vi "Finish.vi"   [LabVIEW 2012]
doc: "This VI is called just before exiting. It is expected to close I/O refnum, save collected data, etc."
uses:
  <vilib>/Rock Robotics/WPI/Joystick/WPI_JoystickGetSetRefNum.vi
  <vilib>/Rock Robotics/WPI/RobotDrive/WPI_RobotDriveGetSetRefNum.vi
types:
  T1 = typedef "WPI_DigitalInputDevRef.ctl" = cluster{"DevStatus":errorcluster, "DIO Channel":T2, "Digital Module":T3}
  T2 = typedef "FPGA_DIOChannel.ctl" = enum8{"DIO 1", "DIO 2", "DIO 3", "DIO 4", "DIO 5", "DIO 6", "DIO 7", "DIO 8", "DIO 9", "DIO 10", "DIO 11", "DIO 12", "DIO 13", "DIO 14", "Invalid"}
  T3 = typedef "FPGA_TypedefDigitalModule.ctl" = enum16{"Digital Module 1", "Digital Module 2"}
  T4 = typedef "WPI_EncoderDevRef.ctl" = cluster{"DevStatus":errorcluster, "EncoderIndex":T5, "CounterIndex":T6, "DistancePerCount":dbl, "Decoding Type":T7}
  T5 = typedef "FPGA_EncoderIdx.ctl" = enum8{"Enc 0", "Enc 1", "Enc 2", "Enc 3", "Invalid"}
  T6 = typedef "FPGA_CounterCtrSystemIndex.ctl" = enum8{"Ctr 0", "Ctr 1", "Ctr 2", "Ctr 3", "Ctr 4", "Ctr 5", "Ctr 6", "Ctr 7", "Invalid"}
  T7 = typedef "WPI_EncoderType.ctl" = enum16{"1x", "2x", "4x"}
  T8 = typedef "WPI_MotorControlDeviceRef.ctl" = cluster{"DeviceStatus":errorcluster, "Type":enum16{"PWM", "CAN"}, "PWM":cluster{"Digital Module":T3, "PWM Channel":T9, "DeadBand":T10}, "CAN":cluster{"Device Number":u8, "Control Mode":T11, "Semaphore":T12, "Max Vout":dbl}, "Invert":bool, "TransformRef":T13, "InvTransformRef":T13}
  T9 = typedef "FPGA_DIOPWMChannel.ctl" = enum8{"PWM 1", "PWM 2", "PWM 3", "PWM 4", "PWM 5", "PWM 6", "PWM 7", "PWM 8", "PWM 9", "PWM 10", "Invalid"}
  T10 = typedef "WPI_PWMDeadband.ctl" = cluster{"Name":string, "maxPositivePwm":i32, "minPositivePwm":i32, "centerPwm":i32, "maxNegativePwm":i32, "minNegativePwm":i32, "angularRange":u16}
  T11 = typedef "WPI_CANJaguar_ControlMode.ctl" = enum8{"Percent VBus", "Current", "Speed", "Position", "Voltage"}
  T12 = typedef "Semaphore RefNum" = refnum<k1>
  T13 = typedef "WPI_PWMTransform_ConPane.ctl" = refnum<vi>
  T14 = typedef "WPI_CompressorDevRef.ctl" = cluster{"DevStatus":errorcluster, "DigitalInputDevRef":T1, "RelayDevRef":T15}
  T15 = typedef "WPI_RelayDevRef.ctl" = cluster{"DevStatus":errorcluster, "Relay Channel":T16, "Digital Module":T3, "Relay Direction":T17}
  T16 = typedef "FPGA_DIORelayChannel.ctl" = enum8{"Relay 1", "Relay 2", "Relay 3", "Relay 4", "Relay 5", "Relay 6", "Relay 7", "Relay 8", "Invalid"}
  T17 = typedef "WPI_RelayDirection.ctl" = enum16{"Both directions", "Forward only", "Reverse only"}
  T18 = typedef "WPI_RobotDriveDevRef.ctl" = cluster{"DevStatus":errorcluster, "Motors[]":T8[], "Square Inputs":bool, "Max Output":dbl, "Isochronous":bool}
  T19 = typedef "WPI_SolenoidDevRef.ctl" = cluster{"DevStatus":errorcluster, "Solenoid Module":T20, "Forward Solenoid Channel":T21, "Reverse Solenoid Channel":T21}
  T20 = typedef "FPGA_TypedefSolenoidModule.ctl" = enum16{"Solenoid Module 1", "Solenoid Module 2"}
  T21 = typedef "WPI_SolenoidChannel.ctl" = enum8{"Solenoid 1", "Solenoid 2", "Solenoid 3", "Solenoid 4", "Solenoid 5", "Solenoid 6", "Solenoid 7", "Solenoid 8", "Invalid"}
  T22 = typedef "WPI_AnalogChannelDevRef.ctl" = cluster{"DevStatus":errorcluster, "Analog Module":T23, "Analog Channel":T24}
  T23 = typedef "FPGA_TypedefAnalogModule.ctl" = enum16{"Analog Module 1", "Analog Module 2"}
  T24 = typedef "FPGA_AIChannel.ctl" = enum8{"AI 1", "AI 2", "AI 3", "AI 4", "AI 5", "AI 6", "AI 7", "AI 8", "Invalid"}
  T25 = typedef "WPI_JoystickDevRef.ctl" = cluster{"Device":T26}
  T26 = typedef "WPI_JoystickDeviceEnum.ctl" = enum16{"USB 1", "USB 2", "USB 3", "USB 4", "Kinect 1", "Kinect 2"}
  T27 = typedef "WPI_CameraDevRef.ctl" = cluster{"Camera Address":string, "CameraStatus":errorcluster, "Acquire Image Notifier":refnum<notifier>}
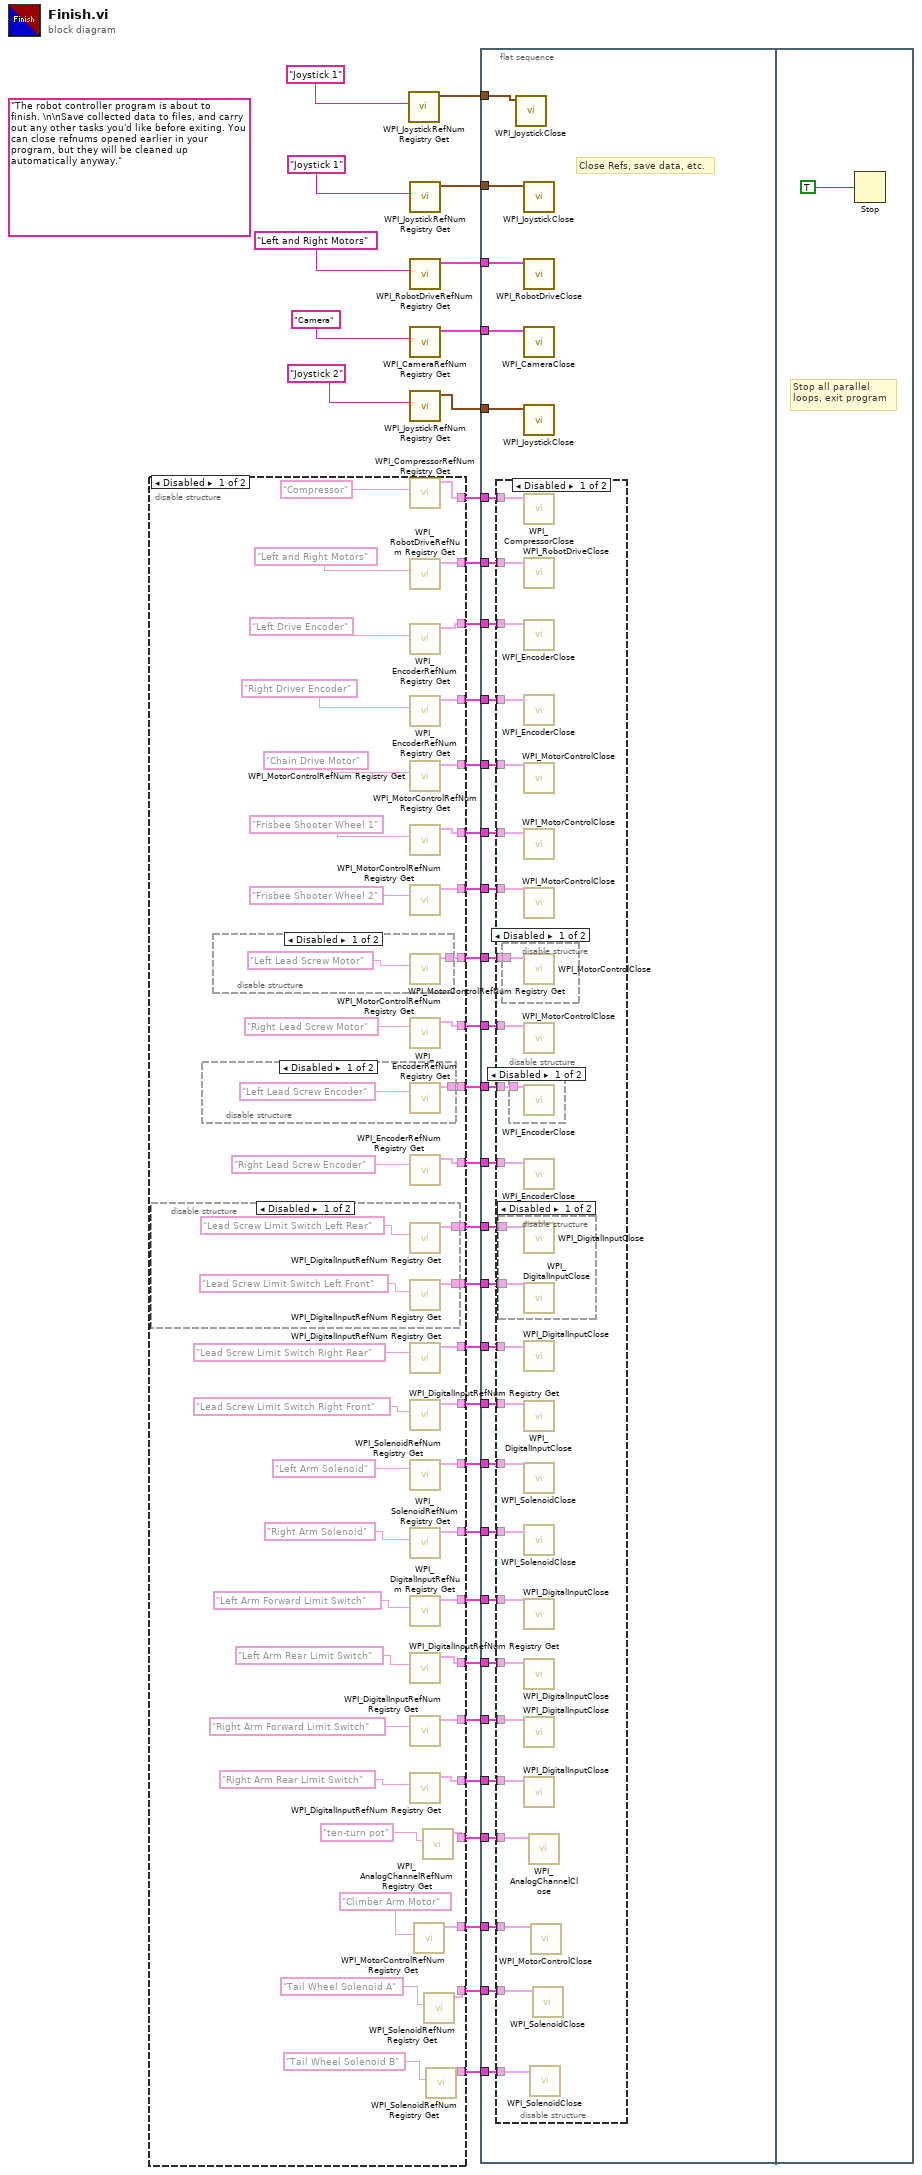
[diagram p0: block diagram]
diagram:
  (unwired) "The robot controller program is about to finish. \n\nSave collected data to files, and carry out any other tasks you'd like before exiting. You can close refnums opened earlier in your program, but they will be cleaned up automatically anyway."
  n1 = disable-structure shown="Disabled" {
    disable-tunnel: [w80 _] -> w27
    disable-tunnel: [w78 _] -> w26
    disable-tunnel: [w75 _] -> w25
    disable-tunnel: [w74 _] -> w24
    disable-tunnel: [w70 _] -> w23
    disable-tunnel: [w69 _] -> w22
    disable-tunnel: [w68 _] -> w21
    disable-tunnel: [w67 _] -> w20
    disable-tunnel: [w66 _] -> w19
    disable-tunnel: [w64 _] -> w18
    disable-tunnel: [w63 _] -> w17
    disable-tunnel: [w59 _] -> w16
    disable-tunnel: [w58 _] -> w15
    disable-tunnel: [w57 _] -> w14
    disable-tunnel: [w56 _] -> w13
    disable-tunnel: [w53 _] -> w12
    disable-tunnel: [w52 _] -> w11
    disable-tunnel: [w51 _] -> w10
    disable-tunnel: [w50 _] -> w9
    disable-tunnel: [w49 _] -> w8
    disable-tunnel: [w48 _] -> w7
    disable-tunnel: [w42 _] -> w4
    disable-tunnel: [w40 _] -> w3
    disable-tunnel: [w37 _] -> w2
    disable-tunnel: [w36 _] -> w1
    frame Disabled {
      n2 = disable-structure shown="Disabled" {
        disable-tunnel: [w87 _] -> w59
        disable-tunnel: [w86 _] -> w58
        frame Disabled {
          n3 = call <vilib>:"WPI_DigitalInputRefNum Registry Get.vi"("refnum name"="Lead Screw Limit Switch Left Rear") -> ("DigitalInputDevRef"=w87:T1)  [unwired: 9 in, 1 out]
          n4 = call <vilib>:"WPI_DigitalInputRefNum Registry Get.vi"("refnum name"="Lead Screw Limit Switch Left Front") -> ("DigitalInputDevRef"=w86:T1)  [unwired: 9 in, 1 out]
        }
        frame Enabled {
        }
      }
      n5 = disable-structure shown="Disabled" {
        disable-tunnel: [w85 _] -> w64
        frame Disabled {
          n6 = call <vilib>:"WPI_EncoderRefNum Registry Get.vi"("refnum name"="Left Lead Screw Encoder") -> ("EncoderDevRef"=w85:T4)  [unwired: 9 in, 1 out]
        }
        frame Enabled {
        }
      }
      n7 = disable-structure shown="Disabled" {
        disable-tunnel: [w83 _] -> w67
        frame Disabled {
          n8 = call <vilib>:"WPI_MotorControlRefNum Registry Get.vi"("refnum name"="Left Lead Screw Motor") -> ("MotorControlDevRef"=w83:T8)  [unwired: 9 in, 1 out]
        }
        frame Enabled {
        }
      }
      n9 = call <vilib>:"WPI_CompressorRefNum Registry Get.vi"("refnum name"="Compressor") -> ("CompressorDevRef"=w80:T14)  [unwired: 9 in, 1 out]
      n10 = call <vilib>:"WPI_RobotDriveRefNum Registry Get.vi"("refnum name"="Left and Right Motors") -> ("RobotDriveDevRef"=w78:T18)  [unwired: 9 in, 1 out]
      n11 = call <vilib>:"WPI_EncoderRefNum Registry Get.vi"("refnum name"="Left Drive Encoder") -> ("EncoderDevRef"=w75:T4)  [unwired: 9 in, 1 out]
      n12 = call <vilib>:"WPI_EncoderRefNum Registry Get.vi"("refnum name"="Right Driver Encoder") -> ("EncoderDevRef"=w74:T4)  [unwired: 9 in, 1 out]
      n13 = call <vilib>:"WPI_MotorControlRefNum Registry Get.vi"("refnum name"="Chain Drive Motor") -> ("MotorControlDevRef"=w70:T8)  [unwired: 9 in, 1 out]
      n14 = call <vilib>:"WPI_MotorControlRefNum Registry Get.vi"("refnum name"="Frisbee Shooter Wheel 1") -> ("MotorControlDevRef"=w69:T8)  [unwired: 9 in, 1 out]
      n15 = call <vilib>:"WPI_MotorControlRefNum Registry Get.vi"("refnum name"="Frisbee Shooter Wheel 2") -> ("MotorControlDevRef"=w68:T8)  [unwired: 9 in, 1 out]
      n16 = call <vilib>:"WPI_MotorControlRefNum Registry Get.vi"("refnum name"="Right Lead Screw Motor") -> ("MotorControlDevRef"=w66:T8)  [unwired: 9 in, 1 out]
      n17 = call <vilib>:"WPI_EncoderRefNum Registry Get.vi"("refnum name"="Right Lead Screw Encoder") -> ("EncoderDevRef"=w63:T4)  [unwired: 9 in, 1 out]
      n18 = call <vilib>:"WPI_DigitalInputRefNum Registry Get.vi"("refnum name"="Lead Screw Limit Switch Right Rear") -> ("DigitalInputDevRef"=w57:T1)  [unwired: 9 in, 1 out]
      n19 = call <vilib>:"WPI_DigitalInputRefNum Registry Get.vi"("refnum name"="Lead Screw Limit Switch Right Front") -> ("DigitalInputDevRef"=w56:T1)  [unwired: 9 in, 1 out]
      n20 = call <vilib>:"WPI_SolenoidRefNum Registry Get.vi"("refnum name"="Left Arm Solenoid") -> ("SolenoidDevRef"=w53:T19)  [unwired: 9 in, 1 out]
      n21 = call <vilib>:"WPI_SolenoidRefNum Registry Get.vi"("refnum name"="Right Arm Solenoid") -> ("SolenoidDevRef"=w52:T19)  [unwired: 9 in, 1 out]
      n22 = call <vilib>:"WPI_DigitalInputRefNum Registry Get.vi"("refnum name"="Left Arm Forward Limit Switch") -> ("DigitalInputDevRef"=w51:T1)  [unwired: 9 in, 1 out]
      n23 = call <vilib>:"WPI_DigitalInputRefNum Registry Get.vi"("refnum name"="Left Arm Rear Limit Switch") -> ("DigitalInputDevRef"=w50:T1)  [unwired: 9 in, 1 out]
      n24 = call <vilib>:"WPI_DigitalInputRefNum Registry Get.vi"("refnum name"="Right Arm Forward Limit Switch") -> ("DigitalInputDevRef"=w49:T1)  [unwired: 9 in, 1 out]
      n25 = call <vilib>:"WPI_DigitalInputRefNum Registry Get.vi"("refnum name"="Right Arm Rear Limit Switch") -> ("DigitalInputDevRef"=w48:T1)  [unwired: 9 in, 1 out]
      n26 = call <vilib>:"WPI_MotorControlRefNum Registry Get.vi"("refnum name"="Climber Arm Motor") -> ("MotorControlDevRef"=w40:T8)  [unwired: 9 in, 1 out]
      n27 = call <vilib>:"WPI_AnalogChannelRefNum Registry Get.vi"("refnum name"="ten-turn pot") -> ("AIDeviceRef"=w42:T22)  [unwired: 9 in, 1 out]
      n28 = call <vilib>:"WPI_SolenoidRefNum Registry Get.vi"("refnum name"="Tail Wheel Solenoid A") -> ("SolenoidDevRef"=w37:T19)  [unwired: 9 in, 1 out]
      n29 = call <vilib>:"WPI_SolenoidRefNum Registry Get.vi"("refnum name"="Tail Wheel Solenoid B") -> ("SolenoidDevRef"=w36:T19)  [unwired: 9 in, 1 out]
    }
    frame Enabled {
    }
  }
  n30 = call <vilib>:"WPI_JoystickRefNum Registry Get.vi"("refnum name"="Joystick 1") -> ("JoystickDevRef"=w5:T25)  [unwired: 1 in, 9 out]
  n31 = call <vilib>:"WPI_JoystickRefNum Registry Get.vi"("refnum name"="Joystick 1") -> ("JoystickDevRef"=w32:T25)  [unwired: 1 in, 9 out]
  n32 = call <vilib>:"WPI_RobotDriveRefNum Registry Get.vi"("refnum name"="Left and Right Motors") -> ("RobotDriveDevRef"=w33:T18)  [unwired: 1 in, 9 out]
  n33 = call <vilib>:"WPI_CameraRefNum Registry Get.vi"("refnum name"="Camera") -> ("CameraDevRef"=w31:T27)  [unwired: 1 in, 9 out]
  n34 = call <vilib>:"WPI_JoystickRefNum Registry Get.vi"("refnum name"="Joystick 2") -> ("JoystickDevRef"=w28:T25)  [unwired: 1 in, 9 out]
  n35 = flat-sequence {
    tunnel: w33 -> [w119]
    tunnel: w32 -> [w118]
    tunnel: w31 -> [w117]
    tunnel: w28 -> [w116]
    tunnel: w27 -> [w115]
    tunnel: w26 -> [w114]
    tunnel: w25 -> [w113]
    tunnel: w24 -> [w112]
    tunnel: w23 -> [w111]
    tunnel: w22 -> [w110]
    tunnel: w21 -> [w109]
    tunnel: w20 -> [w108]
    tunnel: w19 -> [w107]
    tunnel: w18 -> [w106]
    tunnel: w17 -> [w105]
    tunnel: w16 -> [w104]
    tunnel: w15 -> [w103]
    tunnel: w14 -> [w102]
    tunnel: w13 -> [w101]
    tunnel: w12 -> [w100]
    tunnel: w11 -> [w99]
    tunnel: w10 -> [w98]
    tunnel: w9 -> [w97]
    tunnel: w8 -> [w96]
    tunnel: w7 -> [w95]
    tunnel: w5 -> [w94]
    tunnel: w4 -> [w93]
    tunnel: w3 -> [w92]
    tunnel: w2 -> [w91]
    tunnel: w1 -> [w90]
    frame #0 {
      # "Close Refs, save data, etc."
      n36 = disable-structure shown="Disabled" {
        disable-tunnel: w115 -> [w144 _]
        disable-tunnel: w114 -> [w143 _]
        disable-tunnel: w113 -> [w142 _]
        disable-tunnel: w112 -> [w141 _]
        disable-tunnel: w111 -> [w140 _]
        disable-tunnel: w110 -> [w139 _]
        disable-tunnel: w109 -> [w138 _]
        disable-tunnel: w108 -> [w137 _]
        disable-tunnel: w107 -> [w136 _]
        disable-tunnel: w106 -> [w135 _]
        disable-tunnel: w105 -> [w134 _]
        disable-tunnel: w104 -> [w133 _]
        disable-tunnel: w103 -> [w132 _]
        disable-tunnel: w102 -> [w131 _]
        disable-tunnel: w101 -> [w130 _]
        disable-tunnel: w100 -> [w129 _]
        disable-tunnel: w99 -> [w128 _]
        disable-tunnel: w98 -> [w127 _]
        disable-tunnel: w97 -> [w126 _]
        disable-tunnel: w96 -> [w125 _]
        disable-tunnel: w95 -> [w124 _]
        disable-tunnel: w93 -> [w123 _]
        disable-tunnel: w92 -> [w122 _]
        disable-tunnel: w91 -> [w121 _]
        disable-tunnel: w90 -> [w120 _]
        frame Disabled {
          n37 = disable-structure shown="Disabled" {
            disable-tunnel: w133 -> [w148 _]
            disable-tunnel: w132 -> [w147 _]
            frame Disabled {
              n38 = call <vilib>:"WPI_DigitalInputClose.vi"("DigitalInputDevRef"=w148) -> ()  [unwired: 10 in, 1 out]
              n39 = call <vilib>:"WPI_DigitalInputClose.vi"("DigitalInputDevRef"=w147) -> ()  [unwired: 10 in, 1 out]
            }
            frame Enabled {
            }
          }
          n40 = disable-structure shown="Disabled" {
            disable-tunnel: w137 -> [w146 _]
            frame Disabled {
              n41 = call <vilib>:"WPI_MotorControlClose.vi"("MotorControlDevRef"=w146) -> ()  [unwired: 10 in, 1 out]
            }
            frame Enabled {
            }
          }
          n42 = disable-structure shown="Disabled" {
            disable-tunnel: w135 -> [w145 _]
            frame Disabled {
              n43 = call <vilib>:"WPI_EncoderClose.vi"("EncoderDevRef"=w145) -> ()  [unwired: 10 in, 1 out]
            }
            frame Enabled {
            }
          }
          n44 = call <vilib>:"WPI_CompressorClose.vi"("CompressorDevRef"=w144) -> ()  [unwired: 10 in, 1 out]
          n45 = call <vilib>:"WPI_RobotDriveClose.vi"("RobotDriveDevRef"=w143) -> ()  [unwired: 10 in, 1 out]
          n46 = call <vilib>:"WPI_EncoderClose.vi"("EncoderDevRef"=w142) -> ()  [unwired: 10 in, 1 out]
          n47 = call <vilib>:"WPI_EncoderClose.vi"("EncoderDevRef"=w141) -> ()  [unwired: 10 in, 1 out]
          n48 = call <vilib>:"WPI_MotorControlClose.vi"("MotorControlDevRef"=w140) -> ()  [unwired: 10 in, 1 out]
          n49 = call <vilib>:"WPI_MotorControlClose.vi"("MotorControlDevRef"=w139) -> ()  [unwired: 10 in, 1 out]
          n50 = call <vilib>:"WPI_MotorControlClose.vi"("MotorControlDevRef"=w138) -> ()  [unwired: 10 in, 1 out]
          n51 = call <vilib>:"WPI_MotorControlClose.vi"("MotorControlDevRef"=w136) -> ()  [unwired: 10 in, 1 out]
          n52 = call <vilib>:"WPI_EncoderClose.vi"("EncoderDevRef"=w134) -> ()  [unwired: 10 in, 1 out]
          n53 = call <vilib>:"WPI_DigitalInputClose.vi"("DigitalInputDevRef"=w131) -> ()  [unwired: 10 in, 1 out]
          n54 = call <vilib>:"WPI_DigitalInputClose.vi"("DigitalInputDevRef"=w130) -> ()  [unwired: 10 in, 1 out]
          n55 = call <vilib>:"WPI_SolenoidClose.vi"("SolenoidDevRef"=w129) -> ()  [unwired: 10 in, 1 out]
          n56 = call <vilib>:"WPI_SolenoidClose.vi"("SolenoidDevRef"=w128) -> ()  [unwired: 10 in, 1 out]
          n57 = call <vilib>:"WPI_DigitalInputClose.vi"("DigitalInputDevRef"=w127) -> ()  [unwired: 10 in, 1 out]
          n58 = call <vilib>:"WPI_DigitalInputClose.vi"("DigitalInputDevRef"=w126) -> ()  [unwired: 10 in, 1 out]
          n59 = call <vilib>:"WPI_DigitalInputClose.vi"("DigitalInputDevRef"=w125) -> ()  [unwired: 10 in, 1 out]
          n60 = call <vilib>:"WPI_DigitalInputClose.vi"("DigitalInputDevRef"=w124) -> ()  [unwired: 10 in, 1 out]
          n61 = call <vilib>:"WPI_AnalogChannelClose.vi"("AIDeviceRef"=w123) -> ()  [unwired: 10 in, 1 out]
          n62 = call <vilib>:"WPI_SolenoidClose.vi"("SolenoidDevRef"=w120) -> ()  [unwired: 10 in, 1 out]
          n63 = call <vilib>:"WPI_MotorControlClose.vi"("MotorControlDevRef"=w122) -> ()  [unwired: 10 in, 1 out]
          n64 = call <vilib>:"WPI_SolenoidClose.vi"("SolenoidDevRef"=w121) -> ()  [unwired: 10 in, 1 out]
        }
        frame Enabled {
        }
      }
      n65 = call <vilib>:"WPI_JoystickClose.vi"("JoystickDevRef"=w94) -> ()  [unwired: 11 out]
      n66 = call <vilib>:"WPI_JoystickClose.vi"("JoystickDevRef"=w118) -> ()  [unwired: 11 out]
      n67 = call <vilib>:"WPI_RobotDriveClose.vi"("RobotDriveDevRef"=w119) -> ()  [unwired: 1 in, 10 out]
      n68 = call <vilib>:"WPI_CameraClose.vi"("CameraDevRef"=w117) -> ()  [unwired: 1 in, 10 out]
      n69 = call <vilib>:"WPI_JoystickClose.vi"("JoystickDevRef"=w116) -> ()  [unwired: 11 out]
    }
    frame #1 {
      # "Stop all parallel\nloops, exit program"
      n70 = Stop(stop? (T)=TRUE ("Quit")) -> ()
    }
  }
